vi "From MsgPack bytes.vi"(8 "error in (no error)":errorcluster, 10 "Bytes in":u8[](array[numeric]) format="%x", 11 "MessagePack.lvlib:MsgPackExt.lvclass":refnum<class "MsgPackExt.lvclass">) -> (0 "error out":errorcluster, 2 "remaining bytes":u8[](array[numeric]), 3 "MsgPackExt":refnum<class "MsgPackExt.lvclass">)   [LabVIEW 2020, in "MessagePack.lvlib" / "MsgPackExt.lvclass"]
uses:
  MsgPackExt.lvclass
  MsgPackExt.lvclass/MsgPackExt.ctl
  MessagePack.lvlib
  <vilib>/ErrorRing/Error Ring.xnode
  <vilib>/Utility/error.llb/Error Cluster From Error Code.vi
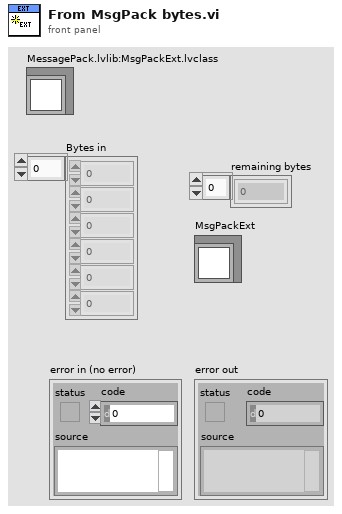
[diagram p1: front panel]
types:
  T1 = typedef "MessagePack.lvlib/MsgPack Object Types.ctl" = enum16{"UNSUPPORTED", "POSINT", "NEGINT", "FIXMAP", "FIXARRAY", "FIXSTR", "NIL", "FALSE", "TRUE", "BIN8", "BIN16", "BIN32", "EXT8", "EXT16", "EXT32", "FLOAT32", "FLOAT64", "UINT8", "UINT16", "UINT32", "UINT64", "INT8", "INT16", "INT32", "INT64", "FIXEXT1", "FIXEXT2", "FIXEXT4", "FIXEXT8", "FIXEXT16", "STR8", "STR16", "STR32", "ARRAY16", "ARRAY32", "MAP16", "MAP32"}
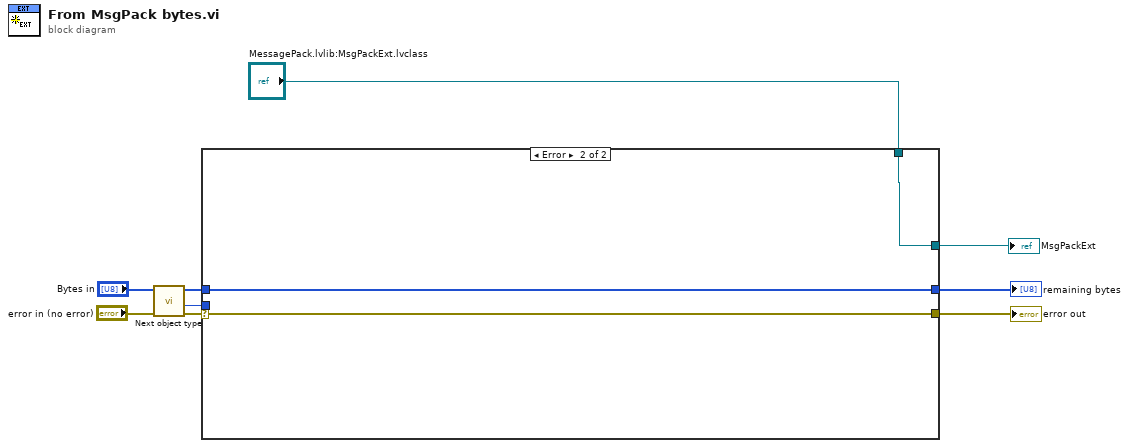
[diagram p0: block diagram]
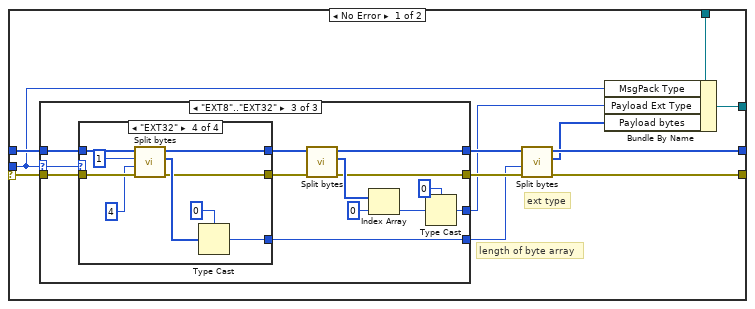
[diagram p2: hidden frame]
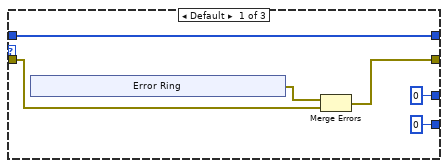
[diagram p3: hidden frame]
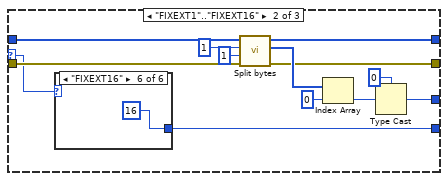
[diagram p4: hidden frame]
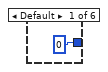
[diagram p5: hidden frame]
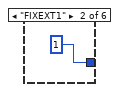
[diagram p6: hidden frame]
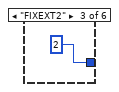
[diagram p7: hidden frame]
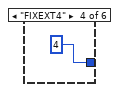
[diagram p8: hidden frame]
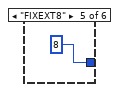
[diagram p9: hidden frame]
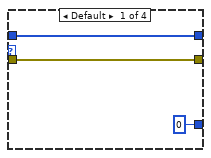
[diagram p10: hidden frame]
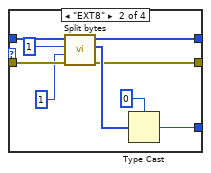
[diagram p11: hidden frame]
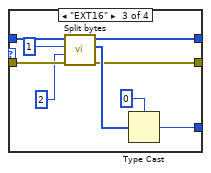
[diagram p12: hidden frame]
diagram:
  n1 = call "Next object type.vi"("error in (no error)"="error in (no error)", "Bytes in"="Bytes in") -> ("error out"=w7:errorcluster, "MsgPack Type"=w6:T1, "Bytes out"=w5:u8[])  [unwired: 6 in, 1 out]
  n2 = case shown="Error" w7 {
    selector: w7 -> [w21 w96]
    tunnel: w6 -> [w11 _]
    tunnel: w5 -> [w20 w95]
    tunnel: [w16 w95] -> w4
    tunnel: [w15 w96] -> w2
    tunnel: [w14 w94] -> w3
    tunnel: "MessagePack.lvlib:MsgPackExt.lvclass" -> [w10 w94]
    frame No Error {
      # "length of byte array"
      # "ext type"
      n3 = case shown="\"EXT8\"..\"EXT32\"" w11 {
        selector: w11 -> [_ w34 w51]
        tunnel: w21 -> [w27 w42 w62]
        tunnel: [w25 w37 w57] -> w18
        tunnel: w20 -> [w24 w44 w63]
        tunnel: [w24 w36 w52] -> w19
        tunnel: [i8 0 w35 w54] -> w13
        tunnel: [u32 0 ("Count") w32 w53] -> w17
        frame Default {
          n4 = xnode "Error Ring"() -> ("error out"=w26:errorcluster)
          n5 = Merge Errors(w26, w27) -> (w25:errorcluster)
        }
        frame "FIXEXT1".."FIXEXT16" {
          n6 = case shown="\"FIXEXT16\"" w34 {
            tunnel: [u32 0 ("Count") u32 1 ("Count") u32 2 ("Count") u32 4 ("Count") u32 8 ("Count") u32 16 ("Count")] -> w32
            frame Default {
            }
            frame "FIXEXT1" {
            }
            frame "FIXEXT2" {
            }
            frame "FIXEXT4" {
            }
            frame "FIXEXT8" {
            }
            frame "FIXEXT16" {
            }
          }
          n7 = call "Split bytes.vi"("error in"=w42, "count (1)"=1 ("Count"), "start index (0)"=1 ("Start index"), "bytes in"=w44) -> ("error out"=w37:errorcluster, "selected bytes"=w40:u8[], "remaining bytes"=w36:u8[])  [unwired: 4 in, 1 out]
          n8 = Index Array(array=w40, index=0) -> (element=w38:u8)
          n9 = Type Cast(type=i8 0, x=w38) -> (*(type *) &x=w35:i8)
        }
        frame "EXT8".."EXT32" {
          n10 = case shown="\"EXT32\"" w51 {
            tunnel: w63 -> [w65 w75 w84 w93]
            tunnel: w62 -> [w66 w73 w82 w91]
            tunnel: [w66 w70 w79 w88] -> w61
            tunnel: [w65 w69 w78 w87] -> w60
            tunnel: [u32 0 w68 w77 w86] -> w53
            frame Default {
            }
            frame "EXT8" {
              n11 = call "Split bytes.vi"("error in"=w73, "count (1)"=1, "start index (0)"=1 ("Start index"), "bytes in"=w75) -> ("error out"=w70:errorcluster, "selected bytes"=w71:u8[], "remaining bytes"=w69:u8[])  [unwired: 4 in, 1 out]
              n12 = Type Cast(type=u8 0, x=w71) -> (*(type *) &x=w68:u8)
            }
            frame "EXT16" {
              n13 = call "Split bytes.vi"("error in"=w82, "count (1)"=2, "start index (0)"=1 ("Start index"), "bytes in"=w84) -> ("error out"=w79:errorcluster, "selected bytes"=w80:u8[], "remaining bytes"=w78:u8[])  [unwired: 4 in, 1 out]
              n14 = Type Cast(type=u16 0, x=w80) -> (*(type *) &x=w77:u16)
            }
            frame "EXT32" {
              n15 = call "Split bytes.vi"("error in"=w91, "count (1)"=4, "start index (0)"=1 ("Start index"), "bytes in"=w93) -> ("error out"=w88:errorcluster, "selected bytes"=w89:u8[], "remaining bytes"=w87:u8[])  [unwired: 4 in, 1 out]
              n16 = Type Cast(type=u32 0, x=w89) -> (*(type *) &x=w86:u32)
            }
          }
          n17 = call "Split bytes.vi"("error in"=w61, "bytes in"=w60) -> ("error out"=w57:errorcluster, "selected bytes"=w59:u8[], "remaining bytes"=w52:u8[])  [unwired: 6 in, 1 out]
          n18 = Index Array(array=w59, index=0) -> (element=w55:u8)
          n19 = Type Cast(type=i8 0, x=w55) -> (*(type *) &x=w54:i8)
        }
      }
      n20 = call "Split bytes.vi"("error in"=w18, "count (1)"=w17, "bytes in"=w19) -> ("error out"=w15:errorcluster, "selected bytes"=w12:u8[], "remaining bytes"=w16:u8[])  [unwired: 5 in, 1 out]
      n21 = Bundle By Name(cluster=w10, "MsgPack Type"=w11, "Payload Ext Type"=w13, "Payload bytes"=w12) -> (w14:refnum<class "MsgPackExt.lvclass">)
    }
    frame Error {
    }
  }
  "error out" <- w2
  "MsgPackExt" <- w3
  "remaining bytes" <- w4
